vi "ReadLog.vi"() -> (3 "data out":T1)   [LabVIEW 2021]
panel:
  in  "Data":T1
  out "error out":errorcluster
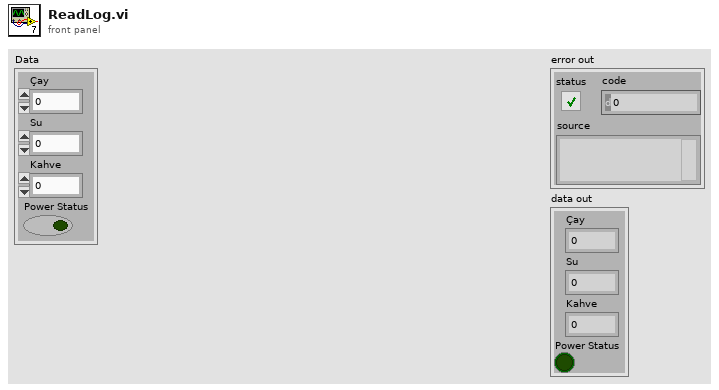
[diagram p1: front panel]
types:
  T1 = cluster{"Çay":dbl, "Su":dbl, "Kahve":dbl, "Power Status":bool}
  T2 = enum16{"open", "replace", "create", "open or create", "replace or create", "replace or create with confirmation"}
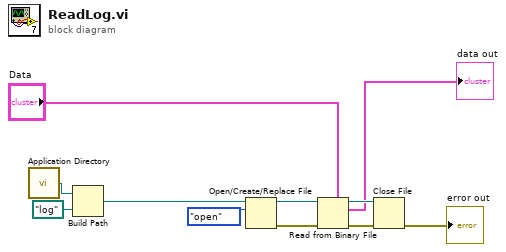
[diagram p0: block diagram]
diagram:
  n1 = call <vilib>:"Application Directory.vi"() -> ("Application Directory"=w7:path)
  n2 = Build Path(base path=w7, name or relative path=path "log") -> (appended path=w4:path)
  n3 = Open/Create/Replace File(file path (use dialog)=w4, operation (0:open)=T2."open") -> (refnum out=w11:refnum<file>, error out=w10:errorcluster)  [unwired: 4 in, 1 out]
  n4 = Read from Binary File(5:"Data", 8:w10, 11:w11) -> (0:w8:errorcluster, 2:→"data out":T1, 3:w9:refnum<file>)  [unwired: 3 in, 1 out]
  n5 = Close File(refnum=w9, error in=w8) -> (error out=→"error out":errorcluster)  [unwired: 1 out]
